vi "Reference Mode Tracking.vi"(0 "Vessel In":refnum<class "Vessel.lvclass">, 1 "x0":dbl[](array[numeric]), 2 "Reset":bool, 3 "u0":dbl[](array[numeric]), 5 "Omega In":T1, 7 "Delta In":T1, 11 "error in":errorcluster, 12 "Position Ref":dbl[](array[numeric])=[0.0, 0.0, 0.0, 0.0, 0.0, 0.0], 13 "Eta_last":dbl[](array[numeric]), 14 "Initialize":bool) -> (4 "Vessel Out":refnum<class "Vessel.lvclass">, 15 "error out":errorcluster)   [LabVIEW 2014]
uses:
  <vilib>/Analysis/Matrix/Datatypes/RealMatrix.ctl
  ROV/Vessel.lvclass
  <vilib>/imath/engines/lvmath2/RunTimeEngine/Managers/WorkSpace/UID Generator.vi
  <vilib>/Analysis/Matrix/Numeric/Conversions/Matrix To Array - RM.vi
  <vilib>/imath/engines/lvmath2/RunTimeEngine/ArithmeticOperatorToken/NIMS_ArithmeticOperator_multmx.vi
  <instcachedir>/0/NIMS_ArithmeticOperator_multmx_CE3986B82B8C4E94A31593A7EF82383B.lvgen/NIMS_ArithmeticOperator_multmx_CE3986B82B8C4E94A31593A7EF82383B_004.vi
  <vilib>/imathl/engines/lvmath/Functions/Error Handling/Create Error.vi
  <vilib>/imath/engines/lvmath2/RunTimeEngine/ArithmeticOperatorToken/NIMS_ArithmeticOperator_plus.vi
  <instcachedir>/0/NIMS_ArithmeticOperator_plus_48D6EAACA5D645B09F7EC9C016C2DEA8.lvgen/NIMS_ArithmeticOperator_plus_48D6EAACA5D645B09F7EC9C016C2DEA8_003.vi
  <instcachedir>/0/NIMS_ArithmeticOperator_plus_48D6EAACA5D645B09F7EC9C016C2DEA8.lvgen/NIMS_ArithmeticOperator_plus_48D6EAACA5D645B09F7EC9C016C2DEA8_012.vi
  <vilib>/imath/engines/lvmath2/RunTimeEngine/ArithmeticOperatorToken/NIMS_ArithmeticOperator_multmx(M,CV).vi
  <instcachedir>/0/NIMS_ArithmeticOperator_multmx(M,CV)_787B4652E60B4C52835A7FB23671E425.lvgen/NIMS_ArithmeticOperator_multmx(M,CV)_787B4652E60B4C52835A7FB23671E425_000.vi
  <vilib>/imath/engines/lvmath2/RunTimeEngine/RunTimeType/NIMS_RunTimeType_From StrictType (excl LVString).vi
  <instcachedir>/0/NIMS_RunTimeType_From StrictType (excl LVString)_15A5391EEA9C4AACB9955AC755B83D29.lvgen/NIMS_RunTimeType_From StrictType (excl LVString)_15A5391EEA9C4AACB9955AC755B83D29_000.vi
  <vilib>/imath/engines/lvmath2/RunTimeEngine/LocalVariableDefStatement/MC_LocalVariableDefStatement_Display.vi
  <vilib>/imath/engines/lvmath2/RunTimeEngine/IndexRead/NIMS M($,S).vi
  <instcachedir>/0/NIMS M($,S)_3E5749BBB62E49528D4765A77F1F6D98.lvgen/NIMS M($,S)_3E5749BBB62E49528D4765A77F1F6D98_000.vi
  <vilib>/imath/engines/lvmath2/RunTimeEngine/ArithmeticOperatorToken/NIMS_ArithmeticOperator_minus.vi
  <instcachedir>/0/NIMS_ArithmeticOperator_minus_39C0593E74DA4138ACA2AB742906488D.lvgen/NIMS_ArithmeticOperator_minus_39C0593E74DA4138ACA2AB742906488D_003.vi
  <vilib>/imath/engines/lvmath2/RunTimeEngine/ErrorHandling/NIMS_Create Error From Enums.vi
  <vilib>/imath/engines/lvmath2/RunTimeEngine/Managers/SymbolTable/Clear UID.vi
  <vilib>/imath/engines/lvmath2/RunTimeEngine/NodeEndStatement/NIMS_NodeEndStatement_Output.vi
  <instcachedir>/0/NIMS_NodeEndStatement_Output_53EC0D466D134D7ABD903AC30B43404B.lvgen/NIMS_NodeEndStatement_Output_53EC0D466D134D7ABD903AC30B43404B_005.vi
  <vilib>/imath/engines/lvmath2/RunTimeEngine/ErrorHandling/NIMS_Finalize Error.vi
  Library/Integrator/Integrator trapez vector.vi
  Library/Kinematics/Jinv_euler.vi
  Library/Kinematics/J_euler.vi
  <vilib>/imath/engines/lvmath2/RunTimeEngine/IndexRead/NIMS M(R2,R2).vi
  <instcachedir>/0/NIMS M(R2,R2)_A604CBC2A3B94D18B31C03B21D5CD7AA.lvgen/NIMS M(R2,R2)_A604CBC2A3B94D18B31C03B21D5CD7AA_000.vi
  <vilib>/imath/engines/lvmath2/RunTimeEngine/IndexRead/NIMS V(R2).vi
  <instcachedir>/0/NIMS V(R2)_C76619605A0E4E9F8B2FA9389712AC47.lvgen/NIMS V(R2)_C76619605A0E4E9F8B2FA9389712AC47_000.vi
  <vilib>/imath/engines/lvmath2/RunTimeEngine/ArithmeticOperatorToken/NIMS_ArithmeticOperator_multmx(M,CV)-internal.vi
  <instcachedir>/0/NIMS_ArithmeticOperator_multmx(M,CV)-internal_25C7CE5937BA4322B5BE2717374345EA.lvgen/NIMS_ArithmeticOperator_multmx(M,CV)-internal_25C7CE5937BA4322B5BE2717374345EA_001.vi
  <vilib>/imath/engines/lvmath2/RunTimeEngine/IndexReplace/NIMS V(R2)=V.vi
  <instcachedir>/0/NIMS V(R2)=V_680A6DA97A4E4BC09213CA62845C7083.lvgen/NIMS V(R2)=V_680A6DA97A4E4BC09213CA62845C7083_000.vi
  <vilib>/imath/engines/lvmath2/RunTimeEngine/IndexRead/NIMS V(S).vi
  <instcachedir>/0/NIMS V(S)_0488751826AF41519A22953C041130DC.lvgen/NIMS V(S)_0488751826AF41519A22953C041130DC_000.vi
  <vilib>/imath/engines/lvmath2/RunTimeEngine/RangeToken/NIMS_Range_R2 - Integer.vi
  <instcachedir>/0/NIMS_Range_R2 - Integer_2D1304BAF97744E0A293025746CBADFC.lvgen/NIMS_Range_R2 - Integer_2D1304BAF97744E0A293025746CBADFC_000.vi
  <vilib>/imath/engines/lvmath2/RunTimeEngine/CommandStatement/MC_CommandStatement_break.vi
  <vilib>/imath/engines/lvmath2/RunTimeEngine/IndexReplace/NIMS V(S)=S.vi
  <instcachedir>/0/NIMS V(S)=S_2D52C4EC15D8415E870AEE69FB516CCA.lvgen/NIMS V(S)=S_2D52C4EC15D8415E870AEE69FB516CCA_000.vi
  <instcachedir>/0/NIMS_NodeEndStatement_Output_53EC0D466D134D7ABD903AC30B43404B.lvgen/NIMS_NodeEndStatement_Output_53EC0D466D134D7ABD903AC30B43404B_002.vi
  <vilib>/Analysis/Matrix/NI_Matrix.lvlib
  <vilib>/imath/engines/lvmath2/RunTimeEngine/Managers/SymbolTable/NIMS_WorkSpace.lvlib
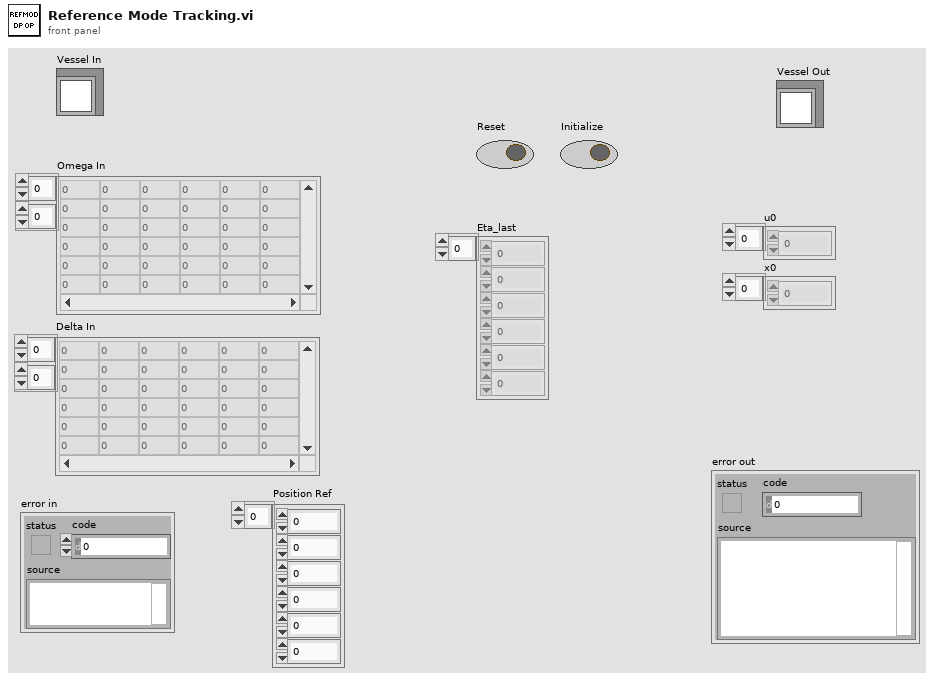
[diagram p1: front panel]
types:
  T1 = typedef "NI_Matrix.lvlib/RealMatrix.ctl" = dbl[][]
  T2 = cluster{"Measured":cluster{"Eta":dbl[], "Nu":dbl[], "Eta Dot":dbl[], "Nu Dot":dbl[]}, "Estimated":cluster{"Eta":dbl[], "Nu":dbl[], "Eta Dot":dbl[], "Nu Dot":dbl[]}, "Desired":cluster{"Eta":dbl[], "Nu":dbl[], "Eta Dot":dbl[], "Nu Dot":dbl[]}, "Previous Desired":cluster{"Eta":dbl[], "Nu":dbl[], "Eta Dot":dbl[], "Nu Dot":dbl[]}, "tau":dbl[], "Altitude":cluster{"Measured":dbl, "Estimated":dbl, "Desired":dbl, "Previous Desired":dbl, "Approximated":dbl, "grad F":dbl[]}, "rpm":dbl[], "Attitude":cluster{"Theta Measured":dbl[], "Theta Estimated":dbl[], "Omega Measured":dbl[], "Omega Estimated":dbl[], "Gyro Bias":dbl[]}}
  T3 = cluster{"Eta":dbl[], "Nu":dbl[], "Eta Dot":dbl[], "Nu Dot":dbl[]}
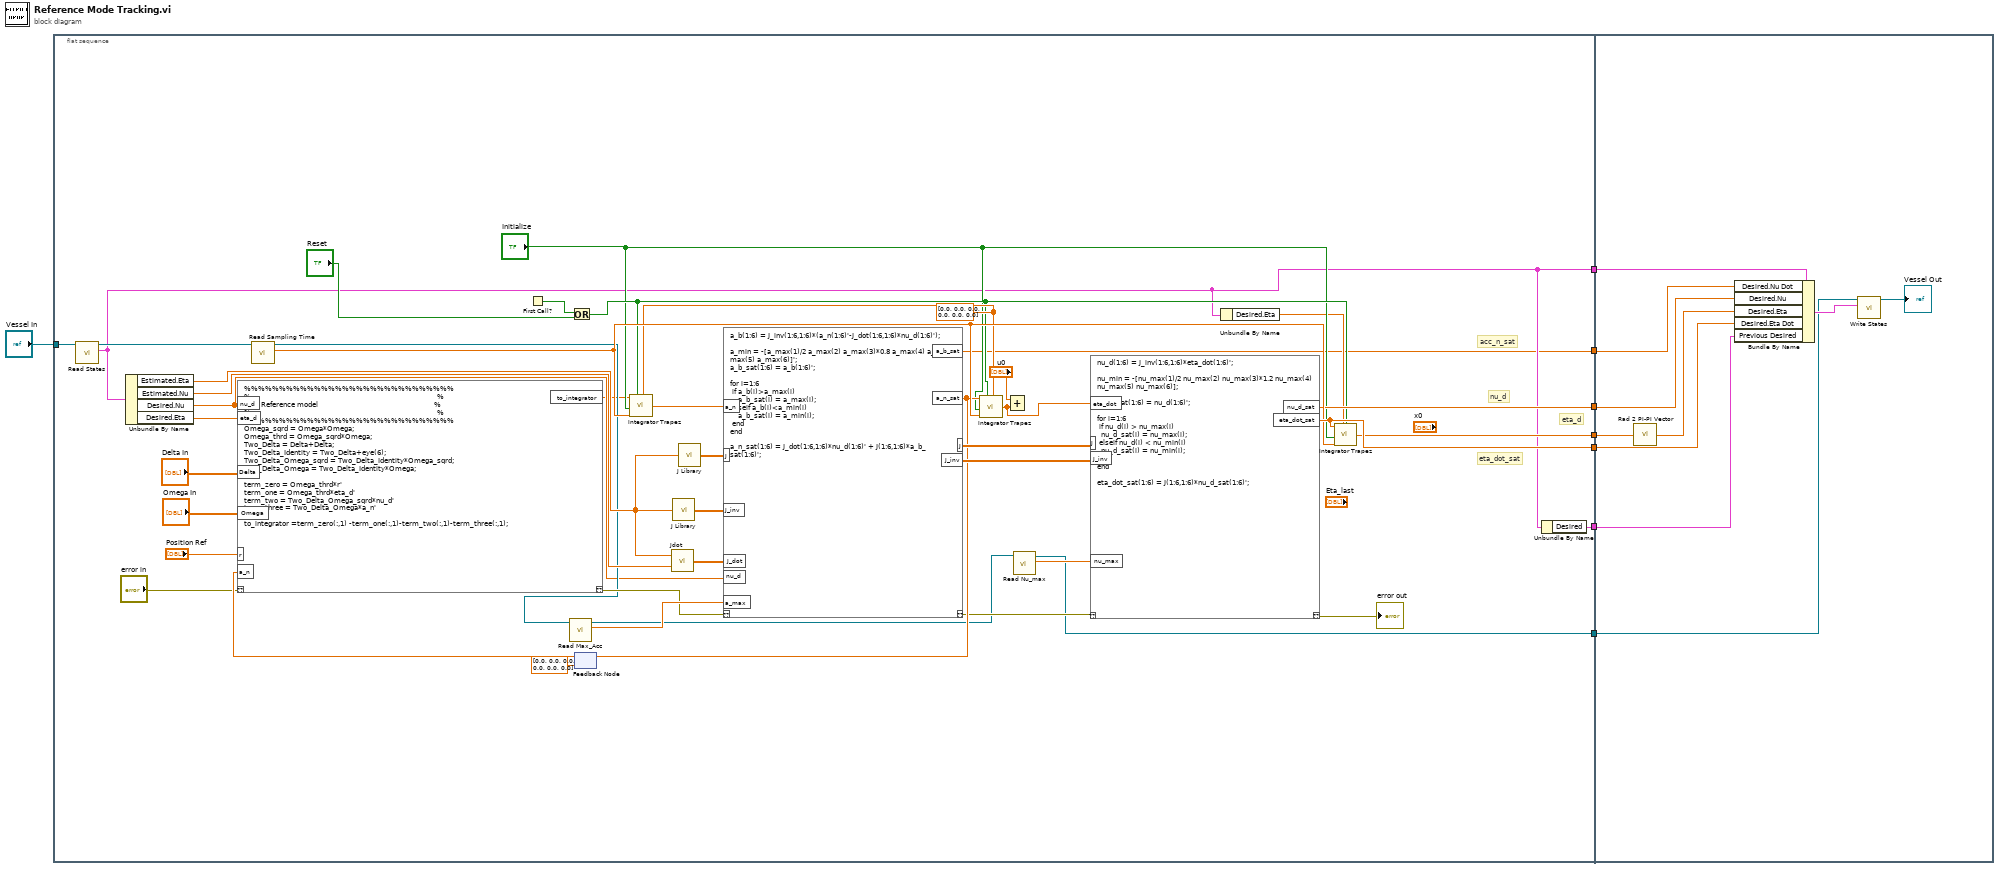
[diagram p0: block diagram]
diagram:
  n1 = flat-sequence {
    tunnel: "Vessel In" -> [w43]
    tunnel: [w12] -> w7
    tunnel: [w41] -> w6
    tunnel: [w21] -> w5
    tunnel: [w15] -> w4
    tunnel: [w14] -> w3
    tunnel: [w29] -> w2
    tunnel: [w23] -> w1
    tunnel: w7 -> [w1137]
    tunnel: w6 -> [w1130]
    tunnel: w5 -> [w1136]
    tunnel: w4 -> [w1132]
    tunnel: w3 -> [w1138]
    tunnel: w2 -> [w1133]
    tunnel: w1 -> [w1129]
    frame #0 {
      w36 = dbl[] [0.0, 0.0, 0.0, 0.0, 0.0, 0.0] ("IC")
      # "acc_n_sat"
      # "eta_dot_sat"
      # "nu_d"
      # "eta_d"
      n2 = call-dynamic "Read States.vi"("Vessel in"=w43) -> ("States"=w14:T2, "Vessel out"=w44:refnum<class "Vessel.lvclass">)  [unwired: 8 in, 1 out]
      n3 = Unbundle By Name(w14) -> ("Estimated.Eta"=w26:dbl[], "Estimated.Nu"=w27:dbl[], "Desired.Nu"=w11:dbl[], "Desired.Eta"=w20:dbl[])
      n4 = call-dynamic "Read Sampling Time.vi"("Vessel in"=w44) -> ("Sampling Time"=w40:dbl, "Vessel out"=w25:refnum<class "Vessel.lvclass">)  [unwired: 8 in, 1 out]
      n5 = First Call?() -> (First Call?: T/F=w19:bool)
      n6 = call "Read Max_Acc.vi"("Vessel in"=w25) -> ("Max_Acc"=w49:dbl[], "Vessel out"=w24:refnum<class "Vessel.lvclass">)  [unwired: 8 in, 1 out]
      n7 = Or(x=w19, y="Reset") -> (x .or. y?=w18:bool)
      n8 = feedback #1(dbl[] [0.0, 0.0, 0.0, 0.0, 0.0, 0.0] ("a_n_sat")) -> (w34:dbl[])
      n9 = mathscript code="%%%%%%%%%%%%%%%%%%%%%%%%%%%%%%\n%                                                                                             %\n%     Reference model                                                          %\n%                                                                                             %\n%%%%%%%%%%%%%%%%%%%%%%%%%%%%%%\nOmega_sqrd = Omega*Omega;\nOmega_thrd = Omega_sqrd*Omega;\nTwo_Delta = Delta+Delta;\nTwo_Delta_Identity = Two_Delta+eye(6);\nTwo_Delta_Omega_sqrd = Two_Delta_Identity*Omega_sqrd;\nTwo_Delta_Omega = Two_Delta_Identity*Omega;\n\nterm_zero = Omega_thrd*r'\nterm_one = Omega_thrd*eta_d'\nterm_two = Two_Delta_Omega_sqrd*nu_d'\nterm_three = Two_Delta_Omega*a_n'\n\nto_integrator =term_zero(:,1) -term_one(:,1)-term_two(:,1)-term_three(:,1);"("??"="error in", "Delta"="Delta In", "Omega"="Omega In", "eta_d"=w20, "nu_d"=w11, "r"="Position Ref", "a_n"=w34) -> ("??"=w33:errorcluster, "to_integrator"=w10:dbl[])
      n10 = call-poly "Integrator Trapez.vi"("IC"=w36, "Reset"=w18, "dt"=w40, "Initialize"="Initialize", "Input"=w10) -> ("Output"=w42:dbl[])  [unwired: 1 in]
      n11 = call "Jdot.vi"("Nu"=w27, "Eta"=w26) -> ("Jdot"=w37:T1)
      n12 = call-poly "J Library.vi"("eta"=w26) -> ("Jinv"=w38:T1)
      n13 = call-poly "J Library.vi"("eta"=w26) -> ("J"=w39:T1)
      n14 = mathscript code="a_b(1:6) = J_inv(1:6,1:6)*(a_n(1:6)'-J_dot(1:6,1:6)*nu_d(1:6)');\n\na_min = -[a_max(1)/2 a_max(2) a_max(3)*0.8 a_max(4) a_max(5) a_max(6)]';\na_b_sat(1:6) = a_b(1:6)';\n\nfor i=1:6\n if a_b(i)>a_max(i)\n    a_b_sat(i) = a_max(i);\n elseif a_b(i)<a_min(i)\n    a_b_sat(i) = a_min(i);\n end \nend\n\na_n_sat(1:6) = J_dot(1:6,1:6)*nu_d(1:6)' + J(1:6,1:6)*a_b_sat(1:6)';"("??"=w33, "a_n"=w42, "nu_d"=w11, "a_max"=w49, "J_inv"=w38, "J_dot"=w37, "J"=w39) -> ("??"=w31:errorcluster, "a_n_sat"=w35:dbl[], "J"=w47:dbl[][], "J_inv"=w46:dbl[][], "a_b_sat"=w12:dbl[])
      n15 = feedback-in #1(w35) -> ()
      n16 = call-poly "Integrator Trapez.vi"("IC"=w36, "Reset"=w18, "dt"=w40, "Initialize"="Initialize", "Input"=w35) -> ("Output"=w9:dbl[])  [unwired: 1 in]
      n17 = Add(x="u0", y=w9) -> ()  [unwired: 1 out]
      n18 = call "Read Nu_max.vi"("Vessel in"=w24) -> ("Nu_max"=w48:dbl[], "Vessel out"=w23:refnum<class "Vessel.lvclass">)  [unwired: 8 in, 1 out]
      n19 = mathscript code="nu_d(1:6) = J_inv(1:6,1:6)*eta_dot(1:6)';\n\nnu_min = -[nu_max(1)/2 nu_max(2) nu_max(3)*1.2 nu_max(4) nu_max(5) nu_max(6)];\n\nnu_d_sat(1:6) = nu_d(1:6)';\n\nfor i=1:6\n if nu_d(i) > nu_max(i)\n  nu_d_sat(i) = nu_max(i);\n elseif nu_d(i) < nu_min(i)\n  nu_d_sat(i) = nu_min(i);\n end\nend\n\neta_dot_sat(1:6) = J(1:6,1:6)*nu_d_sat(1:6)';"("??"=w31, "eta_dot"=w9, "nu_max"=w48, "J"=w47, "J_inv"=w46) -> ("??"=→"error out":errorcluster, "eta_dot_sat"=w41:dbl[], "nu_d_sat"=w21:dbl[])
      n20 = Unbundle By Name(w14) -> ("Desired.Eta"=w13:dbl[])
      n21 = call-poly "Integrator Trapez.vi"("IC"=w13, "Reset"=w18, "dt"=w40, "Initialize"="Initialize", "Input"=w41) -> ("Output"=w15:dbl[])  [unwired: 1 in]
      n22 = Unbundle By Name(w14) -> ("Desired"=w29:T3)
    }
    frame #1 {
      n23 = call "Rad 2 PI-PI Vector.vi"("vector in"=w1132) -> ("vector out"=w1131:dbl[])
      n24 = Bundle By Name(cluster=w1138, "Desired.Nu Dot"=w1137, "Desired.Nu"=w1136, "Desired.Eta"=w1131, "Desired.Eta Dot"=w1130, "Previous Desired"=w1133) -> (w1135:T2)
      n25 = call-dynamic "Write States.vi"("States"=w1135, "Vessel in"=w1129) -> ("Vessel out"=→"Vessel Out":refnum<class "Vessel.lvclass">)  [unwired: 8 in, 1 out]
    }
  }
